vi "Integration Reset.vi"(8 "error in (no error)":errorcluster, 10 "Numeric Control":u8, 11 "Yokogawa WT1600 in":refnum<class "Yokogawa WT1600.lvclass">) -> (0 "error out":errorcluster, 3 "Yokogawa WT1600 out":refnum<class "Yokogawa WT1600.lvclass">)   [LabVIEW 2016, in "Generic Power Analyzer.lvlib" / "Yokogawa WT1600.lvlib" / "Yokogawa WT1600.lvclass"]
uses:
  Yokogawa WT1600.lvclass
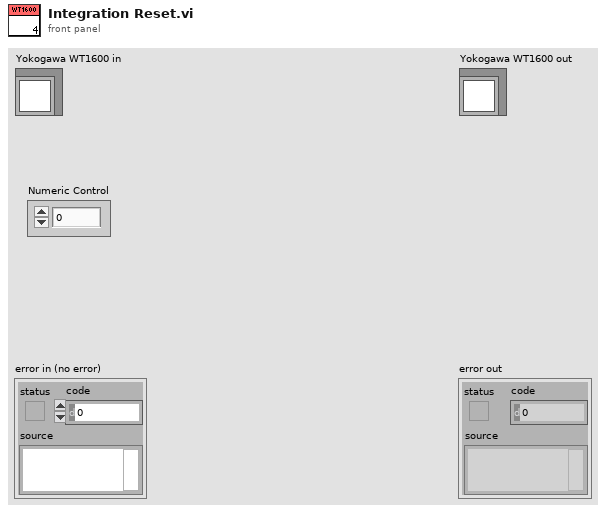
[diagram p1: front panel]
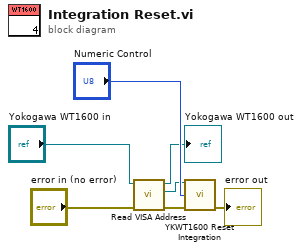
[diagram p0: block diagram]
diagram:
  n1 = call-dynamic "Read VISA Address.vi"("error in (no error)"="error in (no error)", "Generic Device in"="Yokogawa WT1600 in") -> ("error out"=w1:errorcluster, "VISA Address"=w2:refnum<visa-resource-name>, "Generic Device out"=→"Yokogawa WT1600 out":refnum<class "Yokogawa WT1600.lvclass">)  [unwired: 7 in]
  n2 = call <instrlib>:"YKWT1600 Reset Integration.vi"("VISA session"=w2, "Element (All: 0)"="Numeric Control", "error in (no error)"=w1) -> ("error out"=→"error out":errorcluster)  [unwired: 11 in, 1 out]
